vi "InstrEnqueInfront.vi"(1 "Settings":variant, 2 "Para":string caption="Parameter", 3 "PhysCH":string(combo) caption="Physical channel", 4 "Queue in":refnum<queue>) -> (0 "Queue out":refnum<queue>)   [LabVIEW 2017]
uses:
  Action.ctl
  InstrPara.ctl
panel:
  in  "Action":T1
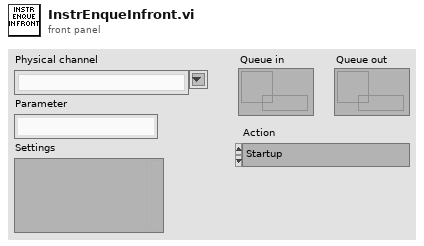
[diagram p1: front panel]
types:
  T1 = typedef "Action.ctl" = enum16{"Startup", "Shutdown", "SaveSettings", "LoadSettings", "InitVNA", "CloseVNA", "InitScan", "IncrementScan", "StopScan", "Target=VNA", "Target=Refrigerator", "Acquire", "Graph", "PNA", "ENA", "ADR", "PPMS"}
  T2 = typedef "InstrPara.ctl" = cluster{"Parameter":string, "Channel":i32, "Instr#":i32, "Settings":variant}
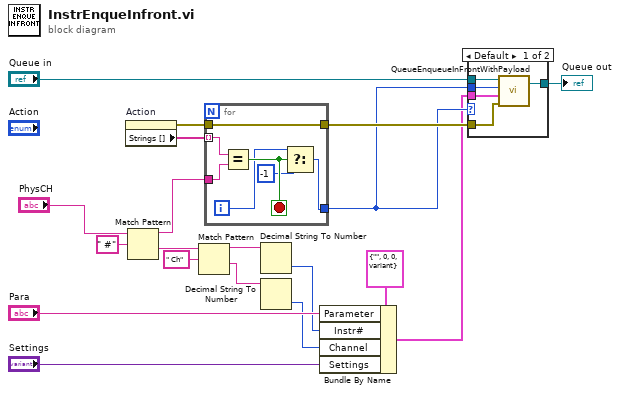
[diagram p0: block diagram]
diagram:
  n1 = property on="Action" class="Enum (strict)"() -> (error out=w6:errorcluster, "Strings []"=w7:string[])  [unwired: 2 in, 1 out]
  n2 = Match Pattern(string="PhysCH", regular expression=" #") -> (before substring=w8:string, after substring=w16:string)  [unwired: 1 in, 2 out]
  n3 = Match Pattern(string=w16, regular expression=" Ch") -> (before substring=w14:string, after substring=w12:string)  [unwired: 1 in, 2 out]
  n4 = for {
    tunnel: w8 -> [w25]
    tunnel: w7 -> [w26] mode=indexing
    tunnel: [w22] -> w4
    tunnel: w6 -> [w24]
    tunnel: [w24] -> w5
    i -> [w21]
    stop <- w23 stop-if-true
    n5 = Equal?(x=w26, y=w25) -> (x = y?=w23:bool)
    n6 = Select(t=w21, s=w23, f=-1) -> (s? t:f=w22:i32)
  }
  n7 = Decimal String To Number(string=w14) -> (number=w13:i32)  [unwired: 2 in, 1 out]
  n8 = Decimal String To Number(string=w12) -> (number=w11:i32)  [unwired: 2 in, 1 out]
  n9 = Bundle By Name(cluster=T2 {"Parameter"="", "Channel"=0, "Instr#"=0, "Settings"=variant(cluster{"Numeric":dbl} {"Numeric"=0.0})} ("Instr. para"), "Parameter"="Para", "Instr#"=w13, "Channel"=w11, "Settings"="Settings") -> (w1:T2)
  n10 = case shown="Default" w4 {
    tunnel: w1 -> [w31 _]
    tunnel: "Queue in" -> [w30 w32]
    tunnel: [w29 w32] -> w9
    tunnel: w4 -> [w28 _]
    tunnel: w5 -> [w27 _]
    frame Default {
      n11 = call "QueueEnqueueInFrontWithPayload.vi"("error in (no error)"=w27, "Payload"=w31, "Action"=w28, "Queue in"=w30) -> ("Queue out"=w29:refnum<queue>)  [unwired: 1 out]
    }
    frame -1 {
    }
  }
  "Queue out" <- w9
